vi "SwerveMath.vi"(0 "X-Axis":dbl, 2 "Y-Axis":dbl, 4 "Turn":dbl) -> (20 "FrontLeftAngle":dbl, 21 "FrontLeftDrive":dbl, 22 "FrontRightAngle":dbl, 23 "FrontRightDrive":dbl, 24 "RearLeftAngle":dbl, 25 "RearLeftDrive":dbl, 26 "RearRightAngle":dbl, 27 "RearRightDrive":dbl)   [LabVIEW 2018]
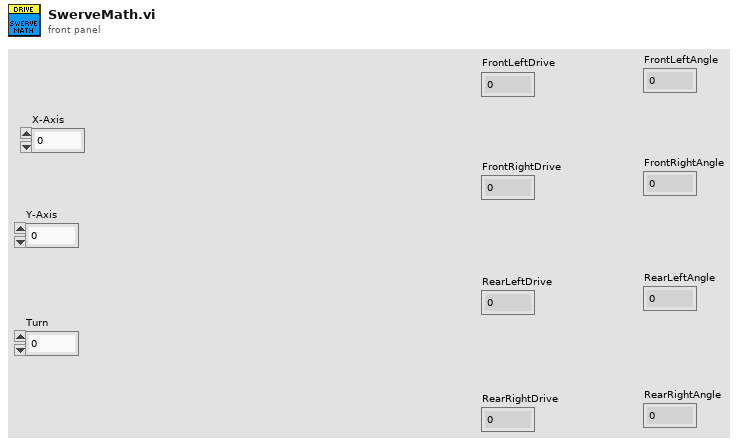
[diagram p1: front panel]
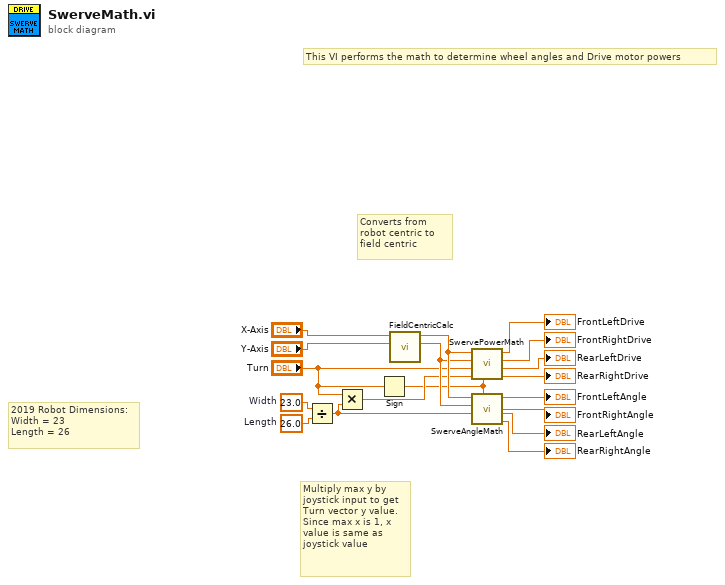
[diagram p0: block diagram]
diagram:
  w17 = 26.0  # Length
  w18 = 23.0  # Width
  # "2019 Robot Dimensions:\nWidth = 23\nLength = 26"
  # "This VI performs the math to determine wheel angles and Drive motor powers"
  # "Converts from robot centric to field centric"
  # "Multiply max y by joystick input to get Turn vector y value.  Since max x is 1, x value is same as joystick value"
  n1 = Divide(x=w18, y=w17) -> (x/y=w3:dbl)
  n2 = Multiply(x="Turn", y=w3) -> (x*y=w8:dbl)
  n3 = Sign(1:"Turn") -> (0:w1:dbl)
  n4 = call "FieldCentricCalc.vi"("y_in"="Y-Axis", "x_in"="X-Axis") -> ("y_out"=w9:dbl, "x_out"=w10:dbl)  [unwired: 8 in]
  n5 = call "SwervePowerMath.vi"("turnSign"=w1, "Turn_y"=w8, "Turn_x"="Turn", "Lateral_y"=w9, "Lateral_x"=w10) -> ("RRDrive"=→"RearRightDrive":dbl, "RLDrive"=→"RearLeftDrive":dbl, "FRDrive"=→"FrontRightDrive":dbl, "FLDrive"=→"FrontLeftDrive":dbl)  [unwired: 3 in]
  n6 = call "SwerveAngleMath.vi"("turnSign"=w1, "whRatio"=w3, "Lateral_y"=w9, "Lateral_x"=w10) -> ("RRAngle"=→"RearRightAngle":dbl, "RLAngle"=→"RearLeftAngle":dbl, "FRAngle"=→"FrontRightAngle":dbl, "FLAngle"=→"FrontLeftAngle":dbl)  [unwired: 4 in]
